vi "Split HeaderTable.vi"(11 "Array (Eingang)":T1[][](array[typedef])) -> (3 "Array (Ausgang)":T1[][](array[typedef]))   [LabVIEW 2020, in "Linearisierung v2.lvlib" / "Protokoll.lvlib"]
uses:
  Protokoll.lvlib
  Visualisierungs Elemente/String - Ausgabefeld.ctl
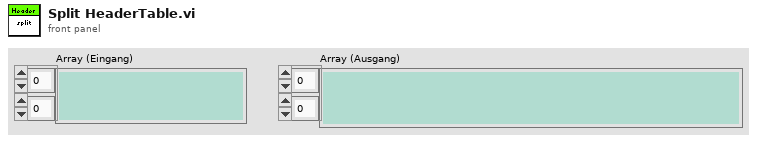
[diagram p1: front panel]
types:
  T1 = typedef "String - Ausgabefeld.ctl" = string
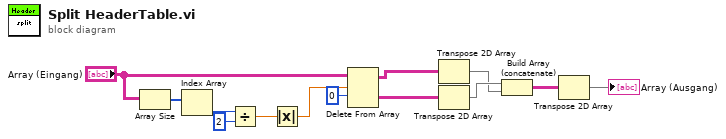
[diagram p0: block diagram]
diagram:
  n1 = Array Size(array="Array (Eingang)") -> (size(s)=w13:i32[])
  n2 = Index Array(array=w13) -> (element=w12:i32)  [unwired: 1 in]
  n3 = Divide(x=w12, y=2) -> (x/y=w10:dbl)
  n4 = Absolute Value(x=w10) -> (abs(x)=w8:dbl)
  n5 = Delete From Array(array="Array (Eingang)", length=w8, index (row)=0 ("Index (Zeile)")) -> (deleted portion=w5:T1[][], array with subset deleted=w6:T1[][])  [unwired: 1 in]
  n6 = Transpose 2D Array(2D array=w6) -> (transposed array=w3:T1[][])
  n7 = Transpose 2D Array(2D array=w5) -> (transposed array=w4:T1[][])
  n8 = Build Array (concatenate)(w4, w3) -> (w2:T1[][])
  n9 = Transpose 2D Array(2D array=w2) -> (transposed array=→"Array (Ausgang)":T1[][])
